vi "Twitter Timestamp to LabVIEW Timestamp.vi"(6 "error in":errorcluster, 9 "Twitter Time Stamp":string="Fri Jul 16 16:40:34 +0000 2010") -> (0 "error out":errorcluster, 3 "LabVIEW Time Stamp":timestamp)   [LabVIEW 2011, in "i3-twitter.lvlib"]
doc: "Convert Twitter timestamp to LabVIEW timestamp."
uses:
  i3-twitter.lvlib
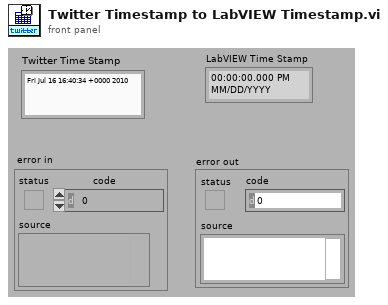
[diagram p1: front panel]
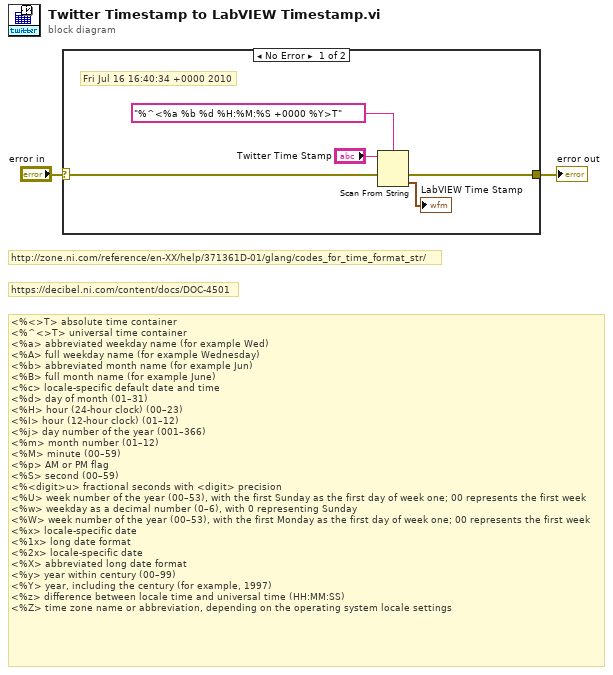
[diagram p0: block diagram]
diagram:
  # "<%<>T>\tabsolute time container\n<%^<>T>\tuniversal time container\n<%a>\tabbreviated weekday name (for example Wed)\n<%A>\tfull weekday name (for example Wednesday)\n<%b>\tabbreviated month name (for example Jun)\n<%B>\tfull month name (for example June)\n<%c>\tlocale-specific default date and time\n<%d>\tday of month (01–31)\n<%H>\thour (24-hour clock) (00–23)\n<%I>\thour (12-hour clock) (01–12)\n<%j>\tday number of the year (001–366)\n<%m>\tmonth number (01–12)\n<%M>\tminute (00–59)\n<%p>\tAM or PM flag\n<%S>\tsecond (00–59)\n<%<digit>u>\tfractional seconds with <digit> precision\n<%U>\tweek number of the year (00–53), with the first Sunday as the first day of week one; 00 represents the first week\n<%w>\tweekday as a decimal number (0–6), with 0 representing Sunday\n<%W>\tweek number of the year (00–53), with the first Monday as the first day of week one; 00 represents the first week\n<%x>\tlocale-specific date\n<%1x>\tlong date format\n<%2x>\tlocale-specific date\n<%X>\tabbreviated long date format\n<%y>\tyear within century (00–99)\n<%Y>\tyear, including the century (for example, 1997)\n<%z>\tdifference between locale time and universal time (HH:MM:SS)\n<%Z>\ttime zone name or abbreviation, depending on the operating system locale settings"
  # "https://decibel.ni.com/content/docs/DOC-4501"
  # "http://zone.ni.com/reference/en-XX/help/371361D-01/glang/codes_for_time_format_str/"
  n1 = case shown="No Error" "error in" {
    selector: "error in" -> [w4 w8]
    tunnel: [w3 w8] -> w1
    frame No Error {
      # "Fri Jul 16 16:40:34 +0000 2010"
      n2 = Scan From String(format string="%^<%a %b %d %H:%M:%S +0000 %Y>T" ("input string"), input string="Twitter Time Stamp", error in=w4) -> (error out=w3:errorcluster, output 1=→"LabVIEW Time Stamp":timestamp)  [unwired: 1 in, 3 out]
    }
    frame Error {
    }
  }
  "error out" <- w1
